vi "onAssertion.vi"(7 "Peel":refnum<class "Project.lvclass">, 10 "Properties":refnum<class "Properties.Assert.lvclass">) -> (0 "error out":errorcluster, 2 "Properties out":refnum<class "Properties.Assert.lvclass">)   [LabVIEW 2021]
uses:
  Project.lvclass
  <vilib>/addons/_JKI Toolkits/Caraya/classes/Properties.Assert/Properties.Assert.lvclass
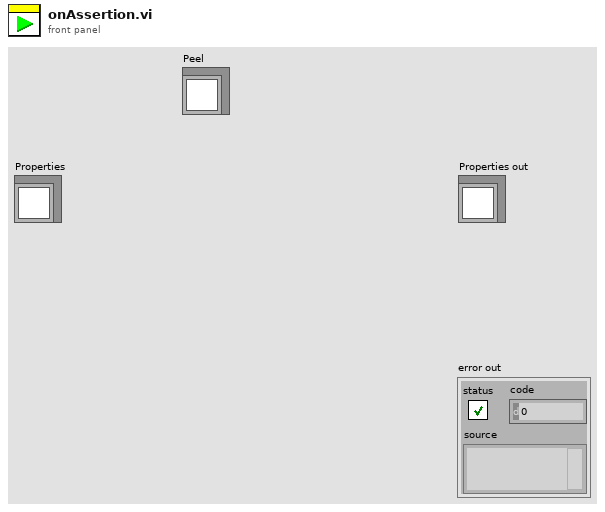
[diagram p1: front panel]
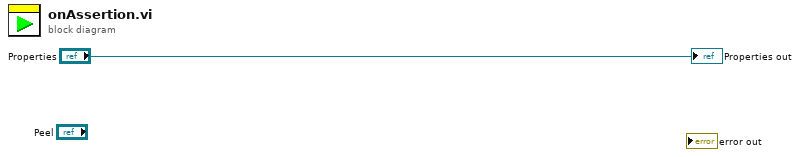
[diagram p0: block diagram]
diagram:
  "Properties out" <- "Properties"
